vi "MeasureBigIV2.vi"(0 ".NET Refnum in":refnum<k24>, 1 ".NET Refnum":refnum<k24>, 2 "Junction Name":string, 7 "appended path":path, 12 "new file path (Not A Path if cancelled)":path, 13 "UiDefinition":T1, 14 "Function":string) -> (15 "error out":errorcluster)   [LabVIEW 2020]
uses:
  D:/LabviewDXFViewer/LabviewDXFViewer/bin/Release/LabviewDXFViewer.exe
  LabviewDXFViewer/bin/Release/LabviewDXFViewer.exe
  UIReferences.ctl
  <vilib>/Analysis/6fits.llb/Curve Fitting Criteria.ctl
  <vilib>/Utility/file.llb/Write Delimited Spreadsheet (string).vi
  <vilib>/Utility/file.llb/Write Delimited Spreadsheet (DBL).vi
  <vilib>/Analysis/NI_AALPro.lvlib
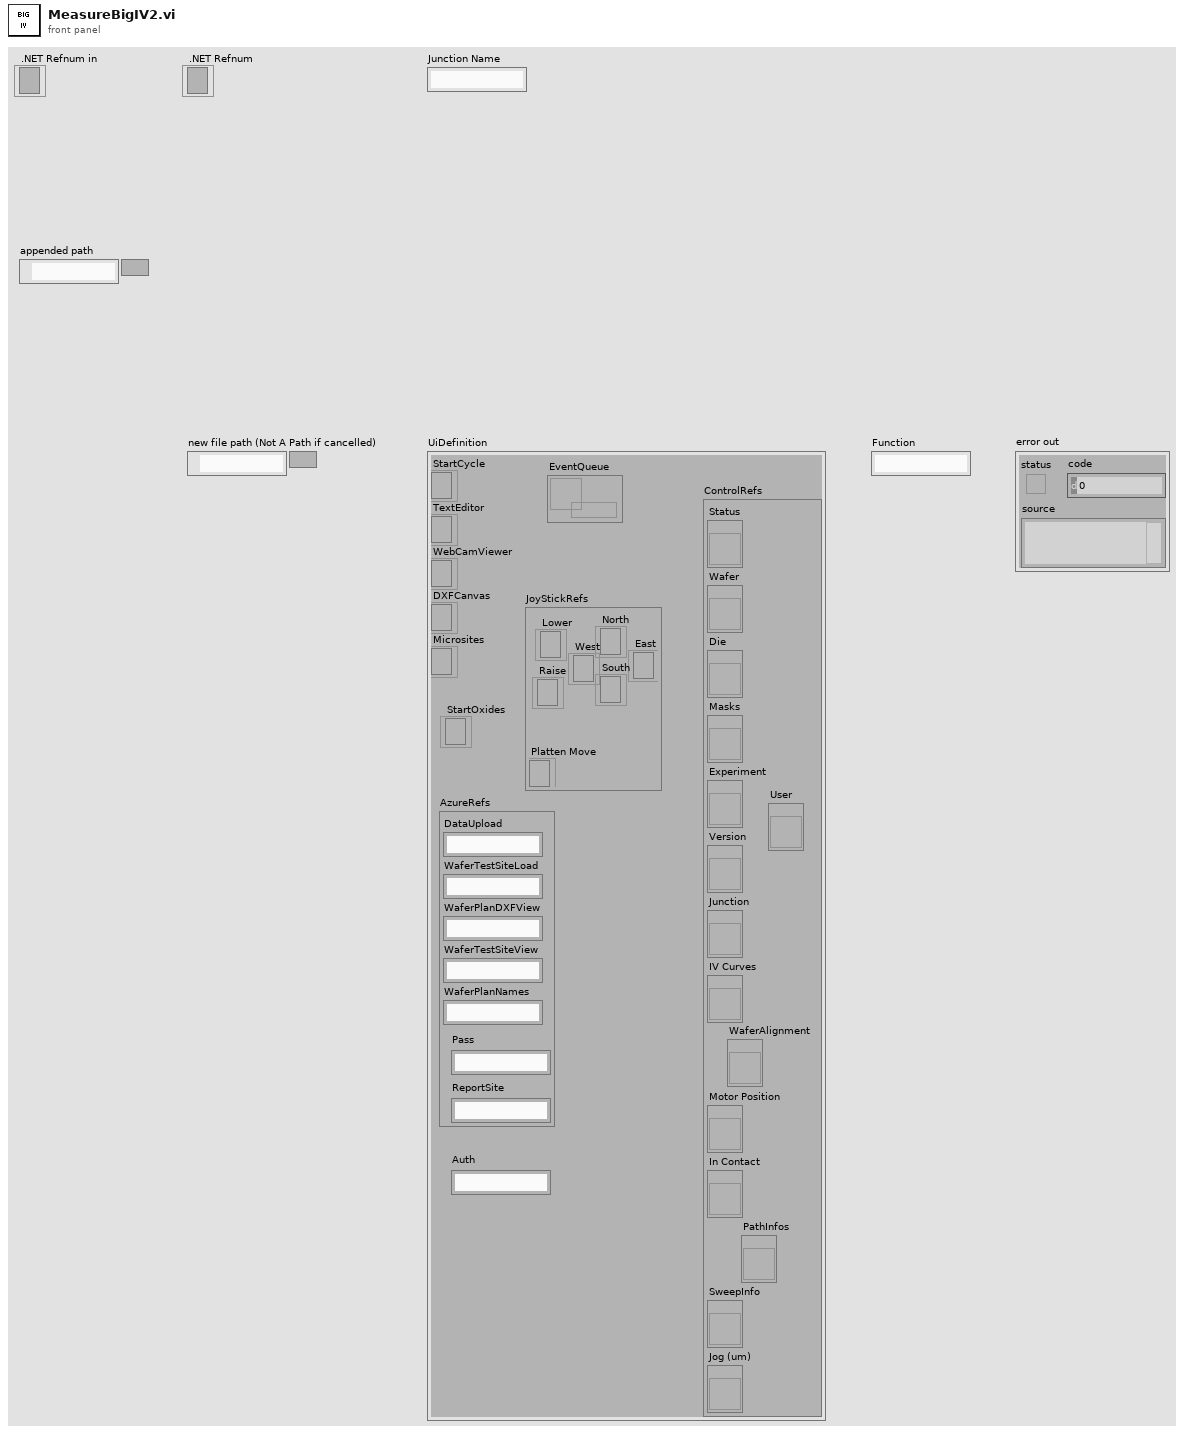
[diagram p1: front panel]
types:
  T1 = typedef "UIReferences.ctl" = cluster{"StartCycle":refnum<k24>, "TextEditor":refnum<k24>, "WebCamViewer":refnum<k24>, "DXFCanvas":refnum<k24>, "Microsites":refnum<k24>, "JoyStickRefs":cluster{"North":refnum<k24>, "Lower":refnum<k24>, "Raise":refnum<k24>, "Platten Move":refnum<k24>, "West":refnum<k24>, "East":refnum<k24>, "South":refnum<k24>}, "AzureRefs":cluster{"DataUpload":string, "WaferTestSiteLoad":string, "WaferPlanDXFView":string, "WaferTestSiteView":string, "WaferPlanNames":string, "Pass":string, "ReportSite":string}, "ControlRefs":cluster{"Status":refnum<vi>, "Wafer":refnum<vi>, "Die":refnum<vi>, "Masks":refnum<vi>, "Experiment":refnum<vi>, "Version":refnum<vi>, "Junction":refnum<vi>, "IV Curves":refnum<vi>, "Motor Position":refnum<vi>, "In Contact":refnum<vi>, "SweepInfo":refnum<vi>, "Jog (um)":refnum<vi>, "PathInfos":refnum<vi>, "User":refnum<vi>, "WaferAlignment":refnum<vi>}, "EventQueue":refnum<queue>, "StartOxides":refnum<k24>, "Auth":string}
  T2 = typedef "NI_AALPro.lvlib/Curve Fitting Criteria.ctl" = u16
  T3 = cluster{"Current Range":dbl, "Source Measure Unit Channel (0: Channel A)":i32, "Waveform":waveform(dbl), "VISA resource name":refnum<visa-resource-name>, "CodeText":string}
  T4 = typedef "CapacitanceInfos.ctl" = cluster{"Conductance":dbl, "CapacitanceIV":dbl, "Intercept":dbl, "CapacitanceSW":dbl, "Sum":dbl, "CapacitanceInfos":T5[], "CapacitancePhase":dbl, "dC/dV":dbl, "Function":string, "OtherInfo":dbl[][], "ChargeCapacitance":dbl, "FitCurves":dbl[][], "Error":dbl, "bestFit":cluster{"Conductance":dbl, "Current0":dbl, "AmpCharge":dbl, "ChargeRC":dbl, "V0":dbl}}
  T5 = typedef "CapacitanceRecord.ctl" = cluster{"Freq":dbl, "Vpp":dbl, "PhaseS":dbl, "Irms":dbl, "PhaseC":dbl, "Theta":dbl, "VDrive":dbl, "Capacitance":dbl, "Other":dbl}
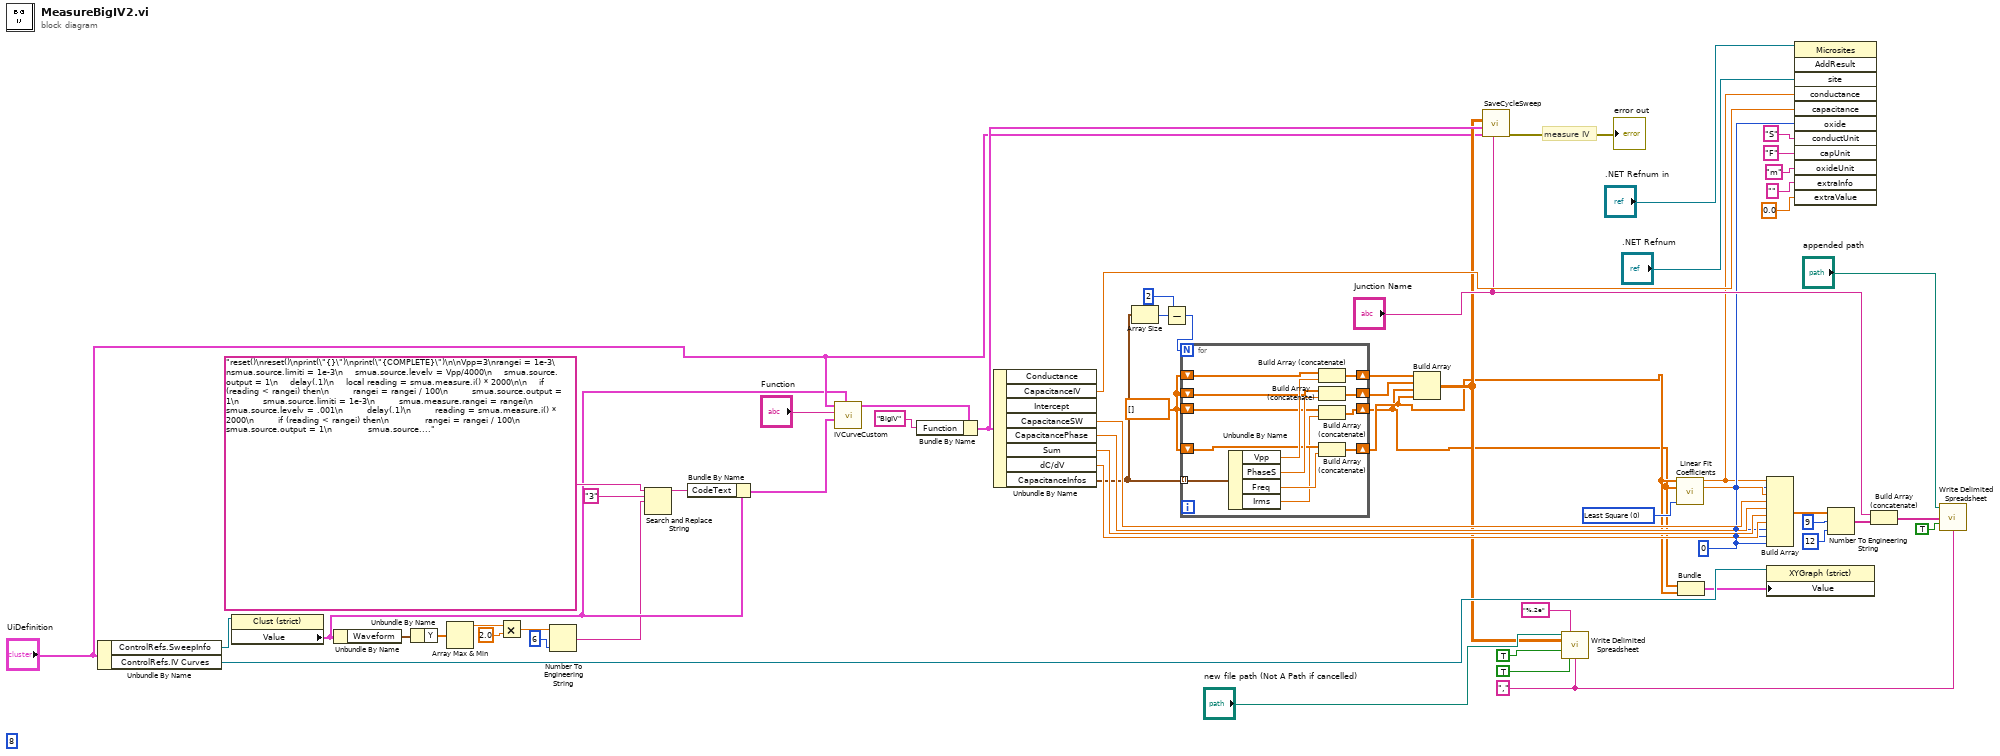
[diagram p0: block diagram]
diagram:
  w8 = 0
  (unwired) i16 8 ("width (-)")
  w26 = T2 0 items=["Least Square", "Least Absolute Residual", "Bisquare"] ("method")
  w30 = dbl[] []
  w37 = "," ("delimiter (\\t)")
  # "measure IV"
  n1 = Unbundle By Name("UiDefinition") -> ("ControlRefs.SweepInfo"=w35:refnum<vi>, "ControlRefs.IV Curves"=w31:refnum<vi>)
  n2 = property class="Clust (strict)"(reference=w35) -> ("Value"=w12:T3)  [unwired: 1 in, 2 out]
  n3 = Unbundle By Name(w12) -> ("Waveform"=w21:waveform(dbl))
  n4 = Unbundle By Name(w21) -> ("Y"=w20:dbl[])
  n5 = Array Max & Min(array=w20) -> (max value=w19:dbl)  [unwired: 3 out]
  n6 = Multiply(x=w19, y=2.0) -> (x*y=w11:dbl)
  n7 = Number To Engineering String(2:i16 6 ("precision (6)"), 4:w11) -> (0:w9:string)  [unwired: 2 in]
  n8 = Search and Replace String(input string="reset()\nreset()\nprint(\"{}\")\nprint(\"{COMPLETE}\")\n\nVpp=3\nrangei = 1e-3\nsmua.source.limiti = 1e-3\n    smua.source.levelv = Vpp/4000\n    smua.source.output = 1\n    delay(.1)\n    local reading = smua.measure.i() * 2000\n\n    if (reading < rangei) then\n        rangei = rangei / 100\n        smua.source.output = 1\n        smua.source.limiti = 1e-3\n        smua.measure.rangei = rangei\n        smua.source.levelv = .001\n        delay(.1)\n        reading = smua.measure.i() * 2000\n        if (reading < rangei) then\n            rangei = rangei / 100\n            smua.source.output = 1\n            smua.source.limiti = 1e-3\n            smua.measure.rangei = rangei\n            smua.source.levelv = .001\n            delay(.1)\n            reading = smua.measure.i() * 2000\n            if (reading < rangei) then\n                rangei = rangei / 1000\n                doCap =1\n                smua.source.levelv = 0\n            end\n        end\n    end\n\nlimitI=rangei\nsmua.source.limiti = rangei\nsmua.source.levelv = Vpp\n\nsmua.source.levelv =0\nsmua.source.output\t\t\t\t\t= smua.OUTPUT_ON\n\n\nVLin=0\nnumCycles=4\nfrequency=2\n\nskips=0\ndisplay=1\n\n\n\tlocal COMPLETE = \"{COMPLETE}\"\n\t-- Generate the source values\n\n\tlocal sourceValues\t\t= {} \n\tlocal pointsPerCycle\t= 60 / frequency\n\tlocal pointsPer60 = 1\n\tlocal numDataPoints\t\t= pointsPerCycle * numCycles\n\n\n\np=pointsPerCycle/2\nlocal x=p/2.0\n    for i = 1, numDataPoints do\n\t    c=math.mod(x,2*p)\n\n        y = Vpp/p*(math.abs(c-p ));\n\n        sourceValues[i] =(y-Vpp/2)\n\nx=x+1\n    end\n\n\t-- Configure the SMU ranges\n\tsmua.reset()\n\tsmua.source.settling\t\t= smua.SETTLE_FAST_POLARITY\n\tsmua.source.autorangev\t\t= smua.AUTORANGE_OFF\n\tsmua.source.autorangei\t\t= smua.AUTORANGE_OFF\n\tsmua.source.rangev\t\t\t=4\n \tsmua.source.limitv\t\t= 2\n\tsmua.source.delay\t\t\t= 0\n\tsmua.source.limiti\t\t\t=1e-3\n\n\tsmua.measure.autorangev\t\t= smua.AUTORANGE_OFF\n\tsmua.measure.autorangei\t\t= smua.AUTORANGE_OFF\n\tsmua.measure.autozero\t\t= smua.AUTOZERO_OFF\n\tsmua.measure.delay\t\t\t= 0\n\tsmua.measure.delayfactor    = 1\n\tsmua.measure.analogfilter   = 0\n\n\t-- Voltage will be measured on the same range as the source range\n\tsmua.measure.rangei\t\t\t=limitI\n\tsmua.measure.nplc\t\t\t=1\n\n\t-- Prepare the Reading Buffers\n\tsmua.nvbuffer1.clear()\n\tsmua.nvbuffer1.collecttimestamps\t= 1\n\tsmua.nvbuffer2.clear()\n\tsmua.nvbuffer2.collecttimestamps\t= 1\n\n\t-- Configure the trigger model\n\t--============================\n\t\n\t-- Timer 1 controls the time between source points\n\ttrigger.timer[1].delay = (1 / 60)\n\ttrigger.timer[1].passthrough = true\n\ttrigger.timer[1].stimulus = smua.trigger.ARMED_EVENT_ID\n\ttrigger.timer[1].count = numDataPoints - 1\n\n\t-- Configure the SMU trigger model\n\tsmua.trigger.source.listv(sourceValues)\n\tsmua.trigger.source.limiti\t\t= limitI\n\tsmua.trigger.measure.action\t\t= smua.ENABLE\n\tsmua.trigger.measure.iv(smua.nvbuffer1, smua.nvbuffer2)\n\tsmua.trigger.endpulse.action\t= smua.SOURCE_HOLD\n\tsmua.trigger.endsweep.action\t= smua.SOURCE_IDLE\n\tsmua.trigger.count\t\t\t\t= numDataPoints\n\tsmua.trigger.arm.stimulus\t\t= 0\n\tsmua.trigger.source.stimulus\t= trigger.timer[1].EVENT_ID\n\tsmua.trigger.measure.stimulus\t= 0\n\tsmua.trigger.endpulse.stimulus\t= 0\n\tsmua.trigger.source.action\t\t= smua.ENABLE\n\t-- Ready to begin the test\n\n\tsmua.source.output\t\t\t\t\t= smua.OUTPUT_ON\n\t-- Start the trigger model execution\n\tsmua.trigger.initiate()\n\t-- Wait until the sweep has completed\n\twaitcomplete()\n\tsmua.source.output\t\t\t\t\t= smua.OUTPUT_OFF\n\n\t-- Print the data back to the Console in tabular format\n\nfor x=1, smua.nvbuffer2.n,pointsPer60 do\n   \n         print(smua.nvbuffer1[x], 1, 1.0/60,smua.nvbuffer1.timestamps[x] ,0 , 0, sourceValues[x],smua.nvbuffer2[x],0)\n    \n\tend\n\nprint(\"{COMPLETE}\")\n\nsmua.source.output = smua.OUTPUT_OFF" ("CodeText"), search string="3", replace string=w9) -> (result string=w17:string)  [unwired: 5 in, 3 out]
  n9 = Bundle By Name(cluster=w12, "CodeText"=w17) -> (w16:T3)
  n10 = call "IVCurveCustom.vi"("OriginalSweepInfo"=w12, "SweepInfo"=w16, "Program"="Function", "UiDefinition"="UiDefinition") -> ("InfoCluster"=w13:T4)  [unwired: 6 in, 1 out]
  n11 = Bundle By Name(cluster=w13, "Function"="BigIV") -> (w34:T4)
  n12 = Unbundle By Name(w34) -> ("CapacitanceIV"=w60:dbl, "CapacitanceSW"=w52:dbl, "CapacitancePhase"=w53:dbl, "Sum"=w50:dbl, "dC/dV"=w51:dbl, "CapacitanceInfos"=w6:T5[])  [unwired: 2 out]
  n13 = Array Size(array=w6) -> (size(s)=w5:i32)
  n14 = Subtract(x=w5, y=2) -> (x-y=w4:i32)
  n15 = for {
    N: w4 -> [_]
    tunnel: w6 -> [w72] mode=indexing
    shift-right: [w73] -> w27
    shift-left: w30 -> [w70]
    shift-right: [w69] -> w29
    shift-left: w30 -> [w68]
    shift-right: [w65] -> w2
    shift-left: w30 -> [w66]
    shift-right: [w63] -> w1
    shift-left: w30 -> [w64]
    n16 = Unbundle By Name(w72) -> ("Vpp"=w71:dbl, "PhaseS"=w67:dbl, "Freq"=w62:dbl, "Irms"=w61:dbl)
    n17 = Build Array (concatenate)(w70, w71) -> (w73:dbl[])
    n18 = Build Array (concatenate)(w68, w67) -> (w69:dbl[])
    n19 = Build Array (concatenate)(w64, w61) -> (w63:dbl[])
    n20 = Build Array (concatenate)(w66, w62) -> (w65:dbl[])
  }
  n21 = Build Array(w27, w29, w1, w2) -> (w28:dbl[][])
  n22 = call "SaveCycleSweep.vi"("JunctionName"="Junction Name", "UiDefinition 2"="UiDefinition", "InfoCluster"=w34, "appended array"=w28) -> ("error out"=→"error out":errorcluster)  [unwired: 7 in]
  n23 = call-poly <vilib>:"Write Delimited Spreadsheet.vi"("file path (dialog if empty)"="new file path (Not A Path if cancelled)", "format (%.3f)"="%.2e", "2D data"=w28, "append to file? (new file:F)"=TRUE, "transpose? (no:F)"=TRUE, "delimiter (\\t)"=w37) -> ()  [unwired: 8 in, 2 out]
  n24 = call <vilib>:"Linear Fit Coefficients.vi"("Y"=w2, "X"=w1, "method"=w26) -> ("slope"=w7:dbl, "intercept"=w25:dbl)  [unwired: 10 in, 1 out]
  n25 = Bundle(w1, w2) -> (w24:cluster{dbl[], dbl[]})  [unwired: 1 in]
  n26 = Build Array(w7, w8, w25, w52, w53, w50, w51, w8, w8, w8) -> (w49:dbl[])
  n27 = property class="XYGraph (strict)"(reference=w31, "Value"=w24) -> ()  [unwired: 1 in, 2 out]
  n28 = invoke class="Microsites" method="AddResult"(reference=".NET Refnum in", "site"=".NET Refnum", "conductance"=w7, "capacitance"=w60, "oxide"=w8, "conductUnit"="S", "capUnit"="F", "oxideUnit"="m" ("interceptUnit"), "extraInfo"="", "extraValue"=0.0) -> ()  [unwired: 2 in, 12 out]
  n29 = Number To Engineering String(2:i16 12 ("precision (6)"), 3:i16 9 ("width (-)"), 4:w49) -> (0:w42:string[])  [unwired: 1 in]
  n30 = Build Array (concatenate)("Junction Name", w42) -> (w44:string[])
  n31 = call-poly <vilib>:"Write Delimited Spreadsheet.vi"("file path (dialog if empty)"="appended path", "1D data"=w44, "append to file? (new file:F)"=TRUE, "delimiter (\\t)"=w37) -> ()  [unwired: 10 in, 2 out]
